vi "Init All.vi"(4 "Not found":refnum<class "CConfig Query.lvclass">, 6 "Found":refnum<class "CConfig Query.lvclass">, 8 "error in (no error)":errorcluster) -> (0 "error out":errorcluster, 3 "Find First Query out":refnum<class "All Query.lvclass">)   [LabVIEW 2013, in "All Query.lvclass"]
doc: "Copyright 2018, Carya Automatisering, Wiebe Walstra."
uses:
  All Query.lvclass
  CConfig Query.lvclass
  Loop Query.lvclass
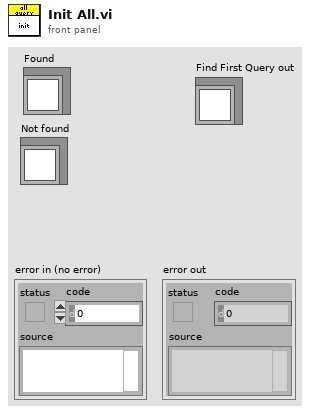
[diagram p1: front panel]
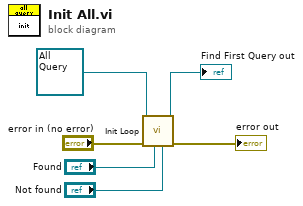
[diagram p0: block diagram]
diagram:
  n1 = call "Init Loop.vi"("Not found"="Not found", "Found"="Found", "error in (no error)"="error in (no error)", "Loop Query"=refnum<class "All Query.lvclass"> refnum ("Find First Query in")) -> ("error out"=→"error out":errorcluster, "Loop Query"=→"Find First Query out":refnum<class "All Query.lvclass">)  [unwired: 6 in]
